vi "Normal_Samples_Generator.vi"(10 "Sampling Info in":T1={"Fs"=10000.0, "#s"=2000.0}, 11 "Number of Normal Samples":i32=10000) -> (3 "data":sgl[][](array[numeric]))   [LabVIEW 2020]
uses:
  Controls/Sampling_Info.ctl
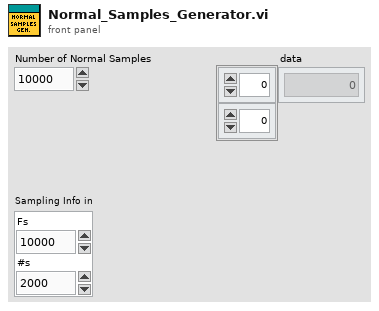
[diagram p1: front panel]
types:
  T1 = typedef "Sampling_Info.ctl" = cluster{"Fs":dbl, "#s":dbl}
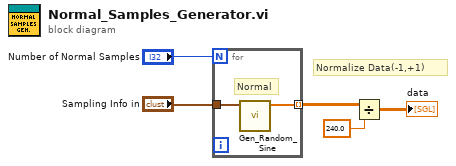
[diagram p0: block diagram]
diagram:
  # "Normalize Data(-1,+1)"
  n1 = for {
    N: "Number of Normal Samples" -> [_]
    tunnel: [w7] -> w2 mode=indexing
    tunnel: "Sampling Info in" -> [w6]
    # "Normal"
    n2 = call "Gen_Random_Sine.vi"("Sampling Info"=w6) -> ("data"=w7:sgl[])  [unwired: 10 in]
  }
  n3 = Divide(x=w2, y=sgl 240.0) -> (x/y=→"data":sgl[][])
